vi "PumpStop.vi"(8 "Error In":errorcluster, 10 "Pump Address":string, 11 "Pump COMM Port":refnum<visa-resource-name>) -> (0 "Error Out":errorcluster)   [LabVIEW 2015]
panel:
  # "Stop Micro Lynx Milligat Pumps"
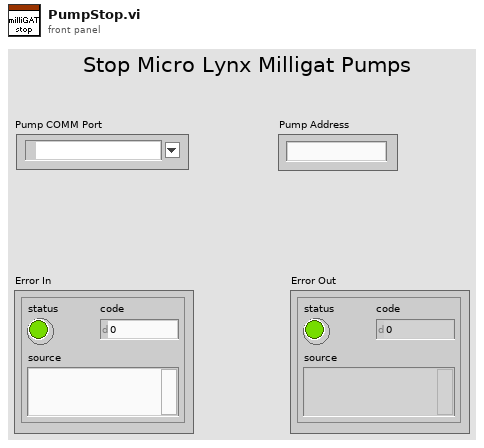
[diagram p1: front panel]
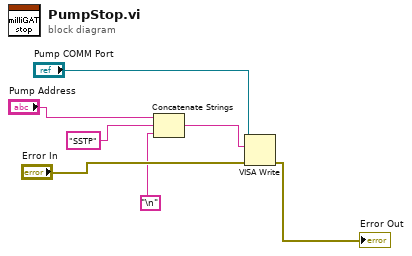
[diagram p0: block diagram]
diagram:
  n1 = Concatenate Strings("Pump Address", "SSTP", "\n") -> (w7:string)
  n2 = VISA Write(VISA resource name="Pump COMM Port", write buffer=w7, error in (no error)="Error In") -> (error out=→"Error Out":errorcluster)  [unwired: 2 out]
